vi "Core-DAQ.vi"(7 "Ctrl-Refs":T1, 8 "Err-I":errorcluster, 9 "ErrQRef":refnum<queue>, 11 "DaqQ-I":refnum<queue>) -> (0 "Err-O":errorcluster)   [LabVIEW 2020]
doc: "DAQ LOOP\nMainly handle the hardware I/O."
uses:
  Core-CtrlRefs.ctl
  <vilib>/drjdpowell/SQLite Library/SQL Statement/SQL Statement.lvclass
  <vilib>/drjdpowell/SQLite Library/SQL Statement/SQL Statement.lvclass/SQL Statement.ctl
  <vilib>/drjdpowell/SQLite Library/SQL Statement/Bind Real.vi
  <vilib>/drjdpowell/SQLite Library/SQL Connection/Open (string).vi
  <vilib>/drjdpowell/SQLite Library/SQL Statement/Step.vi
  <vilib>/AdvancedString/Path To Command Line String.vi
  <vilib>/drjdpowell/SQLite Library/SQL Statement/Error Message.vi
  <vilib>/drjdpowell/SQLite Library/SQL Connection/Connection.lvclass
  <vilib>/drjdpowell/SQLite Library/SQL Connection/Execute SQL (No results).vi
  <vilib>/drjdpowell/SQLite Library/SQL Connection/Open (path).vi
  <vilib>/drjdpowell/SQLite Library/SQLite.lvlib
  <vilib>/drjdpowell/SQLite Library/Transaction Helpers/Transaction.lvlib
  <vilib>/ptbypt/NI_PtbyPt.lvlib
panel:
  # ":: Modularized Parallism Templete ::\n- DAQ Loop -\nby: Techie <HighTechYoung@yahoo.com>\nhttp://www.Vigo-tech.com\nCopyright (C) 2010, Vigo Technologies All Rights Reserved"
  # "Inputs"
  # "Outputs"
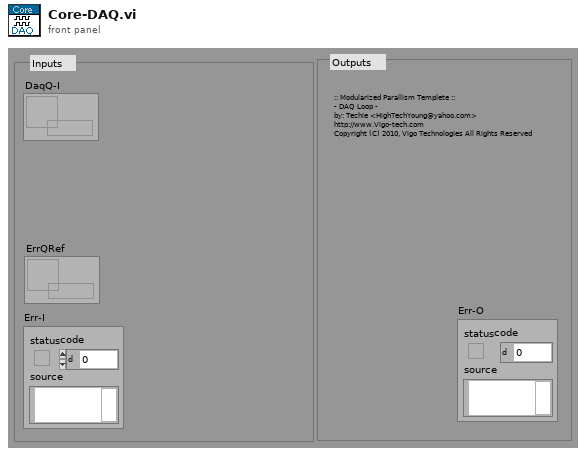
[diagram p1: front panel]
types:
  T1 = typedef "Core-CtrlRefs.ctl" = cluster{"Bool Refnum":refnum<vi>, "DigNum Refnum":refnum<vi>, "WFChart Refnum":refnum<vi>}
  T2 = cluster{"DAQRun?":bool, "SQLite Connection":refnum<class "Connection.lvclass">, "SQL Statement":refnum<class "SQL Statement.lvclass">}
  T3 = cluster{"square wave":dbl, dbl, "Filtered x":dbl}
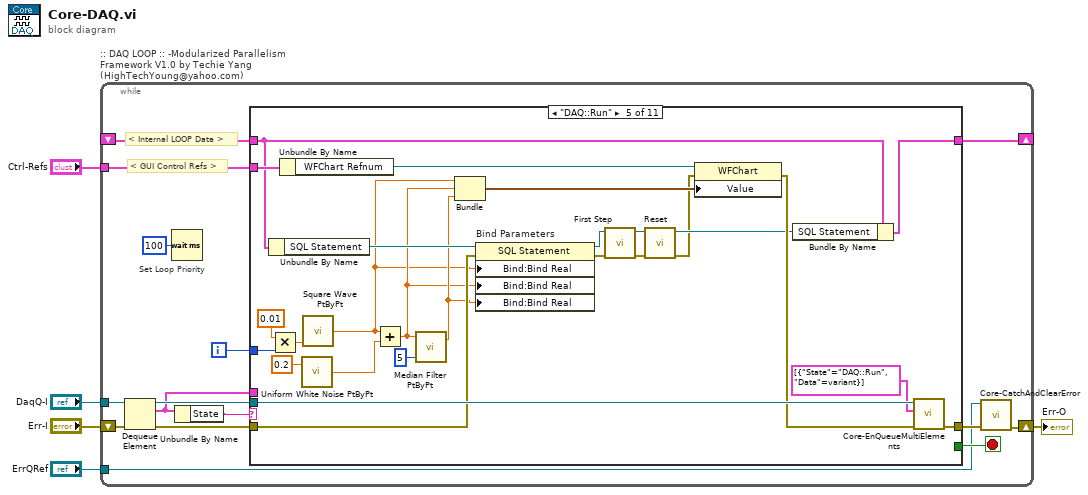
[diagram p0: block diagram]
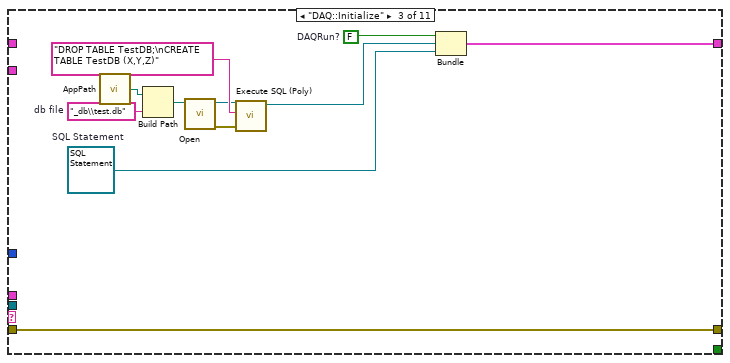
[diagram p4: hidden frame]
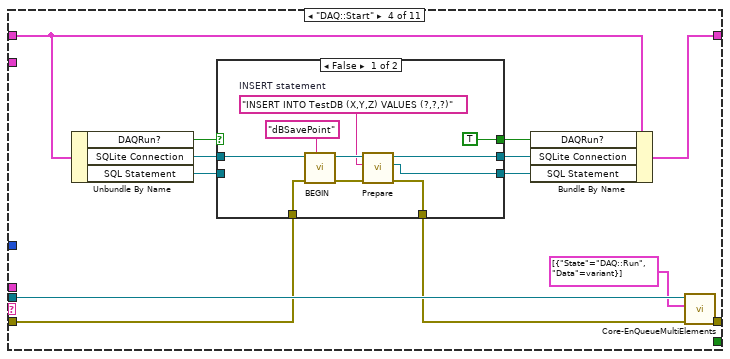
[diagram p5: hidden frame]
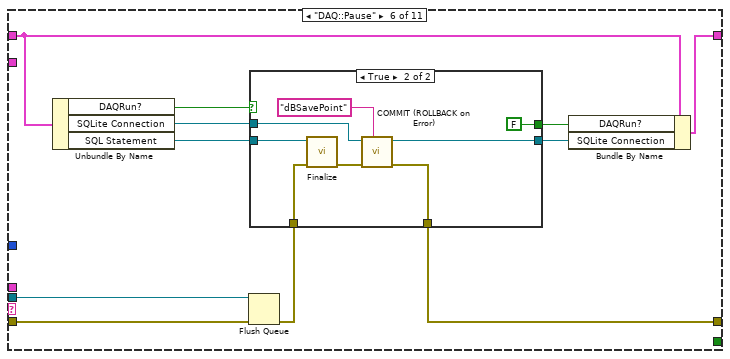
[diagram p7: hidden frame]
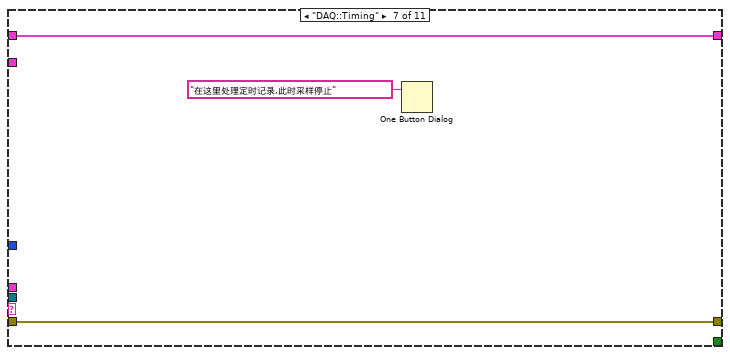
[diagram p9: hidden frame]
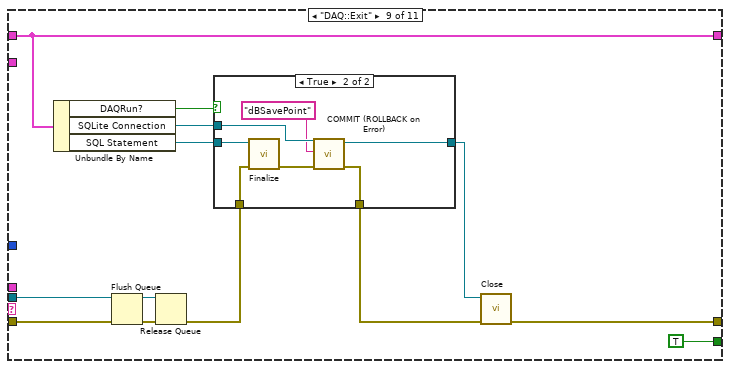
[diagram p11: hidden frame]
diagram:
  n1 = while ":: DAQ LOOP :: -Modularized Parallelism Framework V1.0 by Techie Yang (HighTechYoung@yahoo.com)" {
    tunnel: "DaqQ-I" -> [w20]
    shift-right: [w8] -> w2
    shift-left: "Err-I" -> [w15]
    tunnel: "Ctrl-Refs" -> [w13]
    shift-right: [w12] -> _
    shift-left: _ -> [w11]
    tunnel: "ErrQRef" -> [w7]
    i -> [w6]
    stop <- w18 stop-if-true
    # "Set Loop Priority"
    # "< GUI Control Refs >"
    # "< Internal LOOP Data >"
    n2 = Dequeue Element(queue=w20, error in (no error)=w15) -> (queue out=w17:refnum<queue>, element=w14:cluster{"State":string, "Data":variant}, error out=w19:errorcluster)  [unwired: 2 out]
    n3 = Wait (ms)(milliseconds to wait=u32 100) -> ()  [unwired: 1 out]
    n4 = Unbundle By Name(w14) -> ("State"=w16:string)
    n5 = case shown="\"DAQ::Run\"" w16 {
      tunnel: w19 -> [w21 w24 w34 w45 w73 w98 w113 w114 w127 w139 w141]
      tunnel: [w21 w24 w34 w47 w86 w95 w113 w114 w117 w139 w141] -> w9
      tunnel: [_ _ _ _ _ _ _ _ TRUE _ _] -> w18
      tunnel: w17 -> [_ _ _ w48 w87 w99 _ _ w126 _ _]
      tunnel: w14 -> [_ _ _ _ _ _ _ _ _ _ _]
      tunnel: w13 -> [_ _ _ _ w88 _ _ _ _ _ _]
      tunnel: [w22 w23 w35 w41 w75 w91 w112 w115 w122 w138 w140] -> w12
      tunnel: w11 -> [w22 w23 _ w42 w76 w92 w112 w115 w122 w138 w140]
      tunnel: w6 -> [_ _ _ _ w66 _ _ _ _ _ _]
      frame "IDLE", Default {
      }
      frame "-------- DAQ ---------" {
      }
      frame "DAQ::Initialize" {
        w25 = FALSE  # DAQRun?
        w26 = refnum<class "SQL Statement.lvclass"> refnum  # SQL Statement
        w31 = "_db\\test.db"  # db file
        n6 = call "AppPath.vi"() -> ("AppPath"=w28:path)
        n7 = Build Path(base path=w28, name or relative path=w31) -> (appended path=w29:path)
        n8 = call-poly <vilib>:"Open.vi"("db file"=w29) -> ("error out"=w30:errorcluster, "SQLite Connection"=w32:refnum<class "Connection.lvclass">)  [unwired: 9 in]
        n9 = call-poly <vilib>:"Execute SQL (Poly).vi"("error in (no error)"=w30, "SQL"="DROP TABLE TestDB;\nCREATE TABLE TestDB (X,Y,Z)", "SQLite Connection in"=w32) -> ("SQLite Connection"=w27:refnum<class "Connection.lvclass">)  [unwired: 7 in, 1 out]
        n10 = Bundle("DAQRun?"=w25, "SQLite Connection"=w27, "SQL Statement"=w26) -> (w35:T2)  [unwired: 1 in]
      }
      frame "DAQ::Start" {
        n11 = Unbundle By Name(w42) -> ("DAQRun?"=w38:bool, "SQLite Connection"=w43:refnum<class "Connection.lvclass">, "SQL Statement"=w37:refnum<class "SQL Statement.lvclass">)
        n12 = case shown="False" w38 {
          selector: w38 -> [_ w60]
          tunnel: w45 -> [w55 w59]
          tunnel: [w54 w59] -> w44
          tunnel: w43 -> [w53 w62]
          tunnel: [w51 w62] -> w40
          tunnel: [w50 w61] -> w39
          tunnel: w37 -> [_ w61]
          tunnel: [TRUE w60] -> w36
          frame False {
            w52 = "INSERT INTO TestDB (X,Y,Z) VALUES (?,?,?)"  # INSERT statement
            n13 = call <vilib>:"BEGIN.vi"("Savepoint name"="dBSavePoint", "error in (no error)"=w55, "SQLite Connection in"=w53) -> ("error out"=w57:errorcluster, "SQLite Connection"=w58:refnum<class "Connection.lvclass">)  [unwired: 7 in]
            n14 = call <vilib>:"Prepare.vi"("error in (no error)"=w57, "SQL"=w52, "SQLite Connection in"=w58) -> ("error out"=w54:errorcluster, "SQL Statement"=w50:refnum<class "SQL Statement.lvclass">, "SQLite Connection"=w51:refnum<class "Connection.lvclass">)  [unwired: 4 in, 2 out]
          }
          frame True {
          }
        }
        n15 = Bundle By Name(cluster=w42, "DAQRun?"=w36, "SQLite Connection"=w40, "SQL Statement"=w39) -> (w41:T2)
        n16 = call "Core-EnQueueMultiElements.vi"("ErrorIn"=w44, "CmdArray"=cluster{"State":string, "Data":variant}[] [{"State"="DAQ::Run", "Data"=variant}], "QRefIn"=w48) -> ("ErrorOut"=w47:errorcluster)  [unwired: 8 in]
      }
      frame "DAQ::Run" {
        n17 = Unbundle By Name(w76) -> ("SQL Statement"=w77:refnum<class "SQL Statement.lvclass">)
        n18 = Multiply(x=0.01 ("amplitude"), y=w66) -> (x*y=w68:dbl)
        n19 = Unbundle By Name(w88) -> ("WFChart Refnum"=w83:refnum<vi>)
        n20 = call <vilib>:"Uniform White Noise PtByPt.vi"("amplitude"=0.2) -> ("uniform white noise"=w69:dbl)  [unwired: 2 in]
        n21 = call <vilib>:"Square Wave PtByPt.vi"("time"=w68) -> ("square wave"=w63:dbl)  [unwired: 4 in]
        n22 = Add(x=w63, y=w69) -> (x+y=w64:dbl)
        n23 = call <vilib>:"Median Filter PtByPt.vi"("rank"=5, "x"=w64) -> ("Filtered x"=w65:dbl)  [unwired: 2 in, 1 out]
        n24 = Bundle("square wave"=w63, w64, "Filtered x"=w65) -> (w82:T3)  [unwired: 1 in]
        n25 = property on="Bind Parameters" class="SQL Statement"(reference=w77, error in=w73, "Bind:Bind Real"=w63, "Bind:Bind Real"=w64, "Bind:Bind Real"=w65) -> (reference out=w81:refnum<class "SQL Statement.lvclass">, error out=w80:errorcluster)
        n26 = call <vilib>:"First Step.vi"("error in (no error)"=w80, "SQL Statement in"=w81) -> ("error out"=w79:errorcluster, "SQL Statement"=w78:refnum<class "SQL Statement.lvclass">)  [unwired: 7 in, 1 out]
        n27 = call <vilib>:"Reset.vi"("error in (no error)"=w79, "SQL Statement in"=w78) -> ("error out"=w72:errorcluster, "SQL Statement"=w74:refnum<class "SQL Statement.lvclass">)  [unwired: 8 in]
        n28 = property class="WFChart"(reference=w83, error in=w72, "Value"=w82) -> (error out=w84:errorcluster)  [unwired: 1 out]
        n29 = Bundle By Name(cluster=w76, "SQL Statement"=w74) -> (w75:T2)
        n30 = call "Core-EnQueueMultiElements.vi"("ErrorIn"=w84, "CmdArray"=cluster{"State":string, "Data":variant}[] [{"State"="DAQ::Run", "Data"=variant}], "QRefIn"=w87) -> ("ErrorOut"=w86:errorcluster)  [unwired: 8 in]
      }
      frame "DAQ::Pause" {
        n31 = Unbundle By Name(w92) -> ("DAQRun?"=w90:bool, "SQLite Connection"=w94:refnum<class "Connection.lvclass">, "SQL Statement"=w96:refnum<class "SQL Statement.lvclass">)
        n32 = Flush Queue(queue=w99, error in (no error)=w98) -> (error out=w97:errorcluster)  [unwired: 2 out]
        n33 = case shown="True" w90 {
          selector: w90 -> [w100 _]
          tunnel: w97 -> [w102 w110]
          tunnel: w96 -> [_ w109]
          tunnel: [w102 w107] -> w95
          tunnel: w94 -> [w101 w106]
          tunnel: [w101 w104] -> w93
          tunnel: [w100 FALSE] -> w89
          frame False {
          }
          frame True {
            n34 = call <vilib>:"Finalize.vi"("error in (no error)"=w110, "SQL Statement in"=w109) -> ("error out"=w108:errorcluster)  [unwired: 9 in]
            n35 = call <vilib>:"COMMIT (ROLLBACK on Error).vi"("Savepoint name"="dBSavePoint", "error in (no error)"=w108, "SQLite Connection in"=w106) -> ("error out"=w107:errorcluster, "SQLite Connection"=w104:refnum<class "Connection.lvclass">)  [unwired: 7 in]
          }
        }
        n36 = Bundle By Name(cluster=w92, "DAQRun?"=w89, "SQLite Connection"=w93) -> (w91:T2)
      }
      frame "DAQ::Timing" {
        n37 = One Button Dialog(message="在这里处理定时记录,此时采样停止") -> ()  [unwired: 1 in, 1 out]
      }
      frame "DAQ::UnInitialize" {
      }
      frame "DAQ::Exit" {
        n38 = Unbundle By Name(w122) -> ("DAQRun?"=w116:bool, "SQLite Connection"=w119:refnum<class "Connection.lvclass">, "SQL Statement"=w120:refnum<class "SQL Statement.lvclass">)
        n39 = Flush Queue(queue=w126, error in (no error)=w127) -> (queue out=w124:refnum<queue>, error out=w125:errorcluster)  [unwired: 1 out]
        n40 = Release Queue(queue=w124, error in (no error)=w125) -> (error out=w121:errorcluster)  [unwired: 1 in, 2 out]
        n41 = case shown="True" w116 {
          tunnel: [w130 w137] -> w123
          tunnel: w121 -> [w129 w136]
          tunnel: w120 -> [_ w135]
          tunnel: w119 -> [w130 w133]
          tunnel: [w129 w132] -> w118
          frame False {
          }
          frame True {
            n42 = call <vilib>:"Finalize.vi"("error in (no error)"=w136, "SQL Statement in"=w135) -> ("error out"=w134:errorcluster)  [unwired: 9 in]
            n43 = call <vilib>:"COMMIT (ROLLBACK on Error).vi"("Savepoint name"="dBSavePoint", "error in (no error)"=w134, "SQLite Connection in"=w133) -> ("error out"=w132:errorcluster, "SQLite Connection"=w137:refnum<class "Connection.lvclass">)  [unwired: 7 in]
          }
        }
        n44 = call-dynamic "Close.vi"("error in (no error)"=w118, "SQLite Connection in"=w123) -> ("error out"=w117:errorcluster)  [unwired: 9 in]
      }
      frame "--------User Case---------" {
      }
      frame "Reserved" {
      }
    }
    n45 = call "Core-CatchAndClearError.vi"("Err-I"=w9, "ErrQ-I"=w7) -> ("Err-O"=w8:errorcluster)  [unwired: 9 in]
  }
  "Err-O" <- w2
